vi "Create FIFO Instance String.vi"(9 "Removal Channel":string, 10 "New FIFO Pub":T3 {"New FIFO Instance Config"."Custom Data" format="%.0x"}, 11 "FIFO Publisher":T1 {"FIFO Instance Config"."Custom Data" format="%.0x"}) -> (1 "FIFO Instance info string":string, 3 "FIFO Instance string":string)   [LabVIEW 2021, in "CIFLogs.lvlib"]
uses:
  CIFLogs.lvlib
  CIFCore/Common/Typedef/FIFO Publisher.ctl
  <vilib>/CIF Foundation/CIF Channels Core/ChannelCommon/typedef/New FIFO Instance Configuration.ctl
  Channels/CIFChannelMng/typedef/FIFO Publisher Return.ctl
  <vilib>/CIF Foundation/CIF Channels Core/ChannelCommon/ChannelCommon.lvlib
  CIFCore/Common/CIFCoreCommon.lvlib
  Channels/CIFChannelMng/CIFChannelMng.lvclass
  <vilib>/CIF Foundation/CIF Channels Core/ChannelCommon/typedef/New FIFO Instance Response.ctl
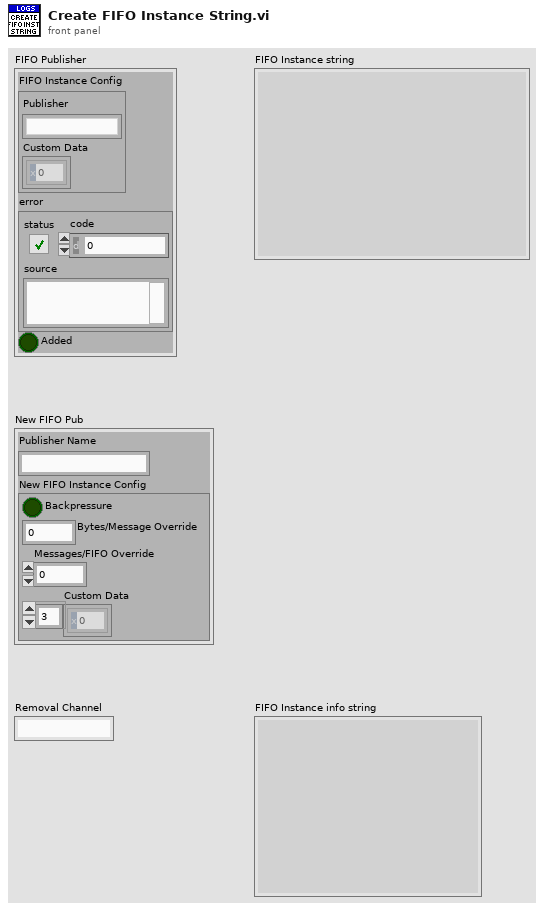
[diagram p1: front panel]
types:
  T1 = typedef "CIFChannelMng.lvclass/FIFO Publisher Return.ctl" = cluster{"FIFO Instance Config":T2, "error":errorcluster, "Added":bool}
  T2 = typedef "ChannelCommon.lvlib/New FIFO Instance Response.ctl" = cluster{"Publisher":string, "Custom Data":u8[]}
  T3 = typedef "CIFCoreCommon.lvlib/FIFO Publisher.ctl" = cluster{"Publisher Name":string, "New FIFO Instance Config":T4}
  T4 = typedef "ChannelCommon.lvlib/New FIFO Instance Configuration.ctl" = cluster{"Backpressure":bool, "Bytes/Message Override":u32, "Messages/FIFO Override":u32, "Custom Data":u8[]}
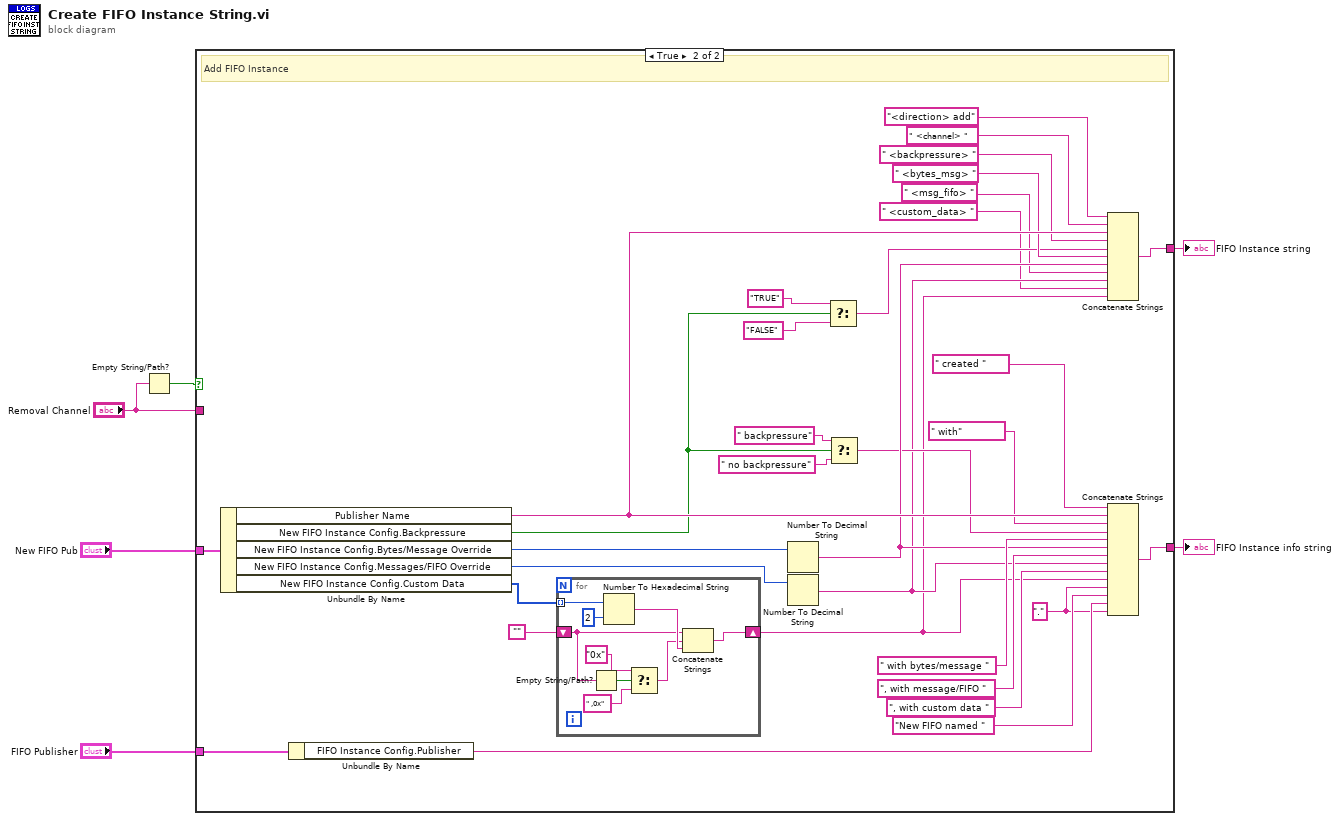
[diagram p0: block diagram]
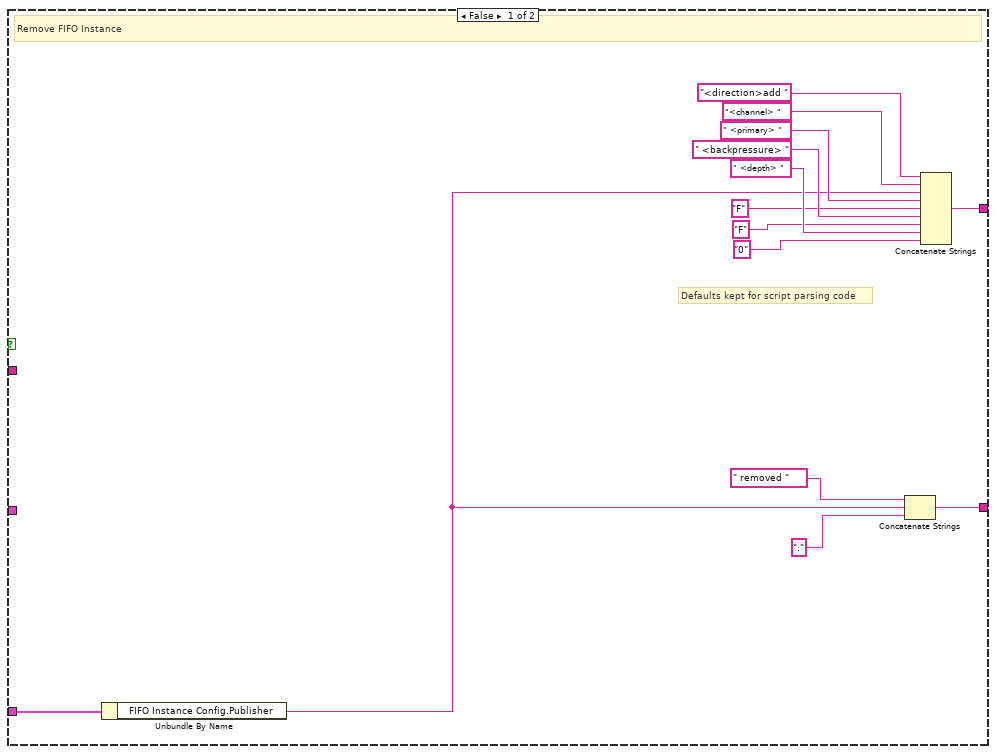
[diagram p2: hidden frame]
diagram:
  n1 = Empty String/Path?(string/path="Removal Channel") -> (empty?=w2:bool)
  n2 = case shown="True" w2 {
    tunnel: [w18 w52] -> w6
    tunnel: [w9 w50] -> w5
    tunnel: "FIFO Publisher" -> [w17 w48]
    tunnel: "New FIFO Pub" -> [_ w47]
    tunnel: "Removal Channel" -> [_ _]
    frame False {
      # "Defaults kept for script parsing code"
      # "Remove FIFO Instance"
      n3 = Unbundle By Name(w17) -> ("FIFO Instance Config.Publisher"=w8:string)
      n4 = Concatenate Strings(" removed " ("string"), w8, "." ("string")) -> (w9:string)
      n5 = Concatenate Strings("<direction>add " ("string"), "<channel> " ("string"), w8, " <primary> " ("string"), "F" ("string"), " <backpressure> " ("string"), "F" ("string"), " <depth> " ("string"), "0" ("string")) -> (w18:string)
    }
    frame True {
      w30 = "." ("string")
      # "Add FIFO Instance"
      n6 = Unbundle By Name(w47) -> ("Publisher Name"=w49:string, "New FIFO Instance Config.Backpressure"=w37:bool, "New FIFO Instance Config.Bytes/Message Override"=w31:u32, "New FIFO Instance Config.Messages/FIFO Override"=w29:u32, "New FIFO Instance Config.Custom Data"=w27:u8[])
      n7 = Unbundle By Name(w48) -> ("FIFO Instance Config.Publisher"=w33:string)
      n8 = for {
        tunnel: w27 -> [w62] mode=indexing
        shift-right: [w56] -> w22
        shift-left: "" -> [w59]
        n9 = Empty String/Path?(string/path=w59) -> (empty?=w61:bool)
        n10 = Number To Hexadecimal String(1:i16 2 ("width (-)"), 2:w62) -> (0:w60:string)
        n11 = Select(t="0x" ("string"), s=w61, f=" ,0x" ("string")) -> (s? t:f=w58:string)
        n12 = Concatenate Strings(w59, w58, w60) -> (w56:string)
      }
      n13 = Number To Decimal String(number=w31) -> (decimal integer string=w46:string)  [unwired: 1 in]
      n14 = Number To Decimal String(number=w29) -> (decimal integer string=w25:string)  [unwired: 1 in]
      n15 = Select(t="TRUE" ("string"), s=w37, f="FALSE" ("string")) -> (s? t:f=w41:string)
      n16 = Select(t=" backpressure" ("string"), s=w37, f=" no backpressure" ("string")) -> (s? t:f=w35:string)
      n17 = Concatenate Strings("<direction> add" ("string"), " <channel> " ("string"), w49, " <backpressure> " ("string"), w41, " <bytes_msg> " ("string"), w46, " <msg_fifo> " ("string"), w25, " <custom_data> " ("string"), w22) -> (w52:string)
      n18 = Concatenate Strings(" created " ("string"), w49, " with" ("string"), w35, " with bytes/message " ("string"), w46, ", with message/FIFO " ("string"), w25, ", with custom data " ("string"), w22, w30, "New FIFO named " ("string"), w33, w30) -> (w50:string)
    }
  }
  "FIFO Instance string" <- w6
  "FIFO Instance info string" <- w5
